vi "generate signal array.vi"(8 "error in":errorcluster, 9 "End":dbl, 10 "Step":dbl, 11 "Start":dbl) -> (0 "error out":errorcluster, 3 "Output":dbl[](array[numeric]))   [LabVIEW 2021]
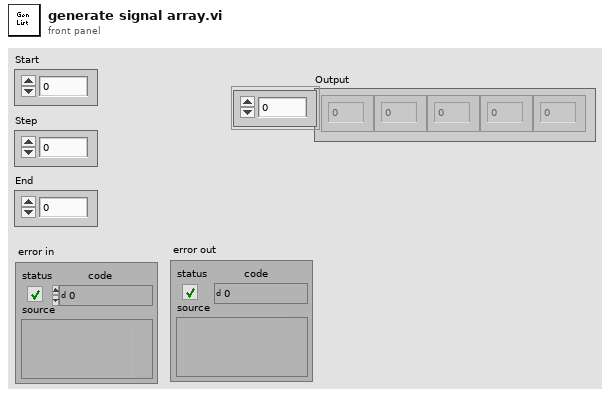
[diagram p1: front panel]
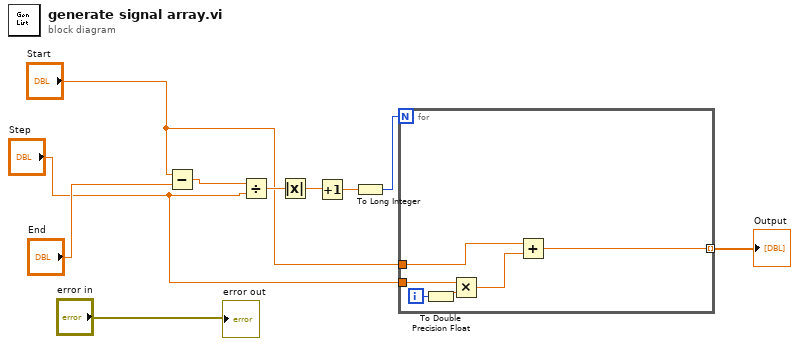
[diagram p0: block diagram]
diagram:
  n1 = Subtract(x="Start", y="End") -> (x-y=w8:dbl)
  n2 = Divide(x=w8, y="Step") -> (x/y=w7:dbl)
  n3 = Absolute Value(x=w7) -> (abs(x)=w6:dbl)
  n4 = Increment(x=w6) -> (x+1=w5:dbl)
  n5 = To Long Integer(number=w5) -> (32bit integer=w4:i32)
  n6 = for {
    N: w4 -> [_]
    tunnel: "Start" -> [w16]
    tunnel: "Step" -> [w12]
    tunnel: [w11] -> w1 mode=indexing
    i -> [w14]
    n7 = To Double Precision Float(number=w14) -> (double precision float=w13:dbl)
    n8 = Multiply(x=w12, y=w13) -> (x*y=w15:dbl)
    n9 = Add(x=w16, y=w15) -> (x+y=w11:dbl)
  }
  "Output" <- w1
  "error out" <- "error in"
